vi "Clear Subpanel.vi"(8 "error in (no error)":errorcluster, 11 "Protected Subpanel":T1) -> (0 "error out":errorcluster, 3 "Protected Subpanel Out":T1)   [LabVIEW 2015, in "IViewable.lvlib" / "ProtectedSubpanel.lvclass"]
uses:
  ProtectedSubpanel.lvclass
  Protected Subpanel Reference.ctl
  ProtectedSubpanel.lvclass/ProtectedSubpanel.ctl
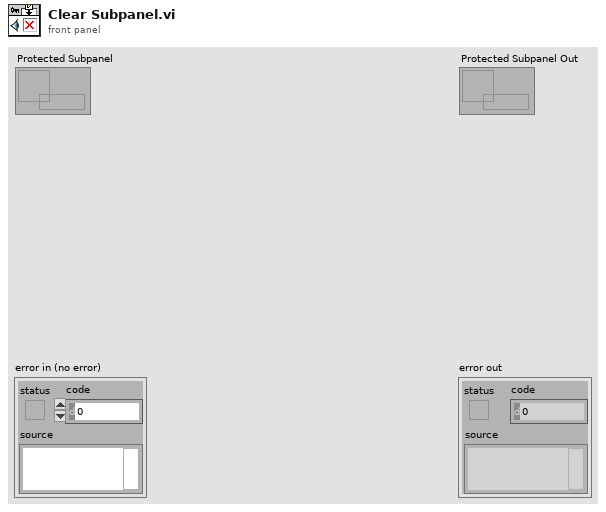
[diagram p1: front panel]
types:
  T1 = typedef "IViewable.lvlib/ProtectedSubpanel.lvclass/Protected Subpanel Reference.ctl" = refnum<data-value>
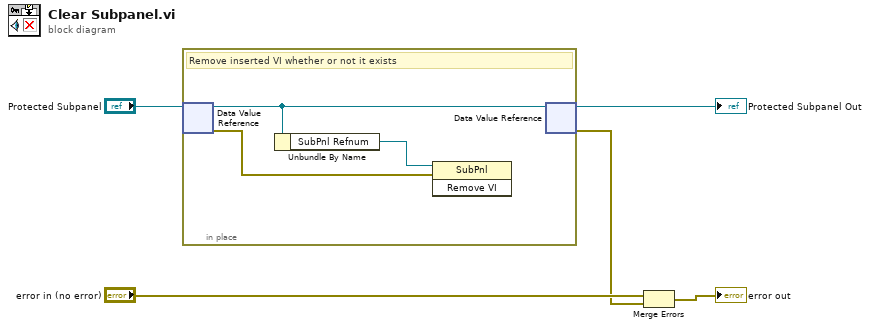
[diagram p0: block diagram]
diagram:
  n1 = in-place {
    # "Remove inserted VI whether or not it exists"
    n2 = in-place-dvr #1("Protected Subpanel") -> (w8:refnum<class "ProtectedSubpanel.lvclass">, w6:errorcluster)
    n3 = Unbundle By Name(w8) -> ("SubPnl Refnum"=w7:refnum<vi>)
    n4 = invoke class="SubPnl" method="Remove VI"(reference=w7, error in=w6) -> ()  [unwired: 1 in, 3 out]
    n5 = in-place-dvr #1(w8) -> (→"Protected Subpanel Out":T1, w1:errorcluster)
  }
  n6 = Merge Errors("error in (no error)", w1) -> (→"error out":errorcluster)
